vi "Get All Available Hardware.vi"(8 "error in (no error)":errorcluster, 11 "Controller in":refnum<class "Controller.lvclass">) -> (0 "error out":errorcluster, 2 "all Hardware in System":refnum<class "Hardware.lvclass">[](array[class]), 3 "Controller out":refnum<class "Controller.lvclass">)   [LabVIEW 2026, in "Controller Actor.lvlib" / "Controller.lvclass"]
uses:
  Controller.lvclass
  Controller.lvclass/Controller.ctl
  Hardware/Hardware.lvclass
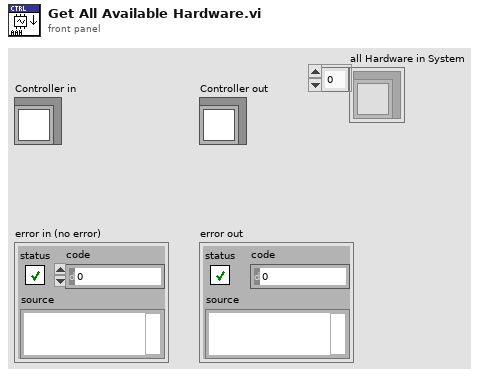
[diagram p1: front panel]
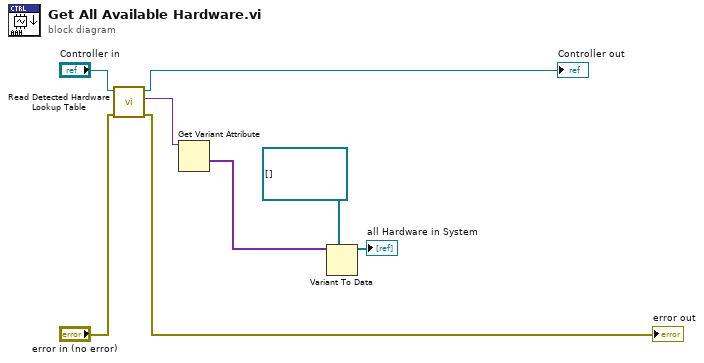
[diagram p0: block diagram]
diagram:
  n1 = call "Read Detected Hardware Lookup Table.vi"("error in (no error)"="error in (no error)", "Controller in"="Controller in") -> ("error out"=→"error out":errorcluster, "Detected Hardware Lookup Table"=w3:variant, "Controller out"=→"Controller out":refnum<class "Controller.lvclass">)  [unwired: 7 in]
  n2 = Get Variant Attribute(Variant=w3) -> (values=w4:variant[])  [unwired: 3 in, 3 out]
  n3 = Variant To Data(type=refnum<class "Hardware.lvclass">[] [], Variant=w4) -> (data=→"all Hardware in System":refnum<class "Hardware.lvclass">[])  [unwired: 1 in, 1 out]
